vi "M03 Hybrid Car.vi"(11 "EV3 in":T1) -> (1 "Angle out":sgl, 3 "EV3 out":T1)   [LabVIEW 2016]
uses:
  <vilib>/NXT/Subs/LVHSConnector.ctl
  <vilib>/NXT/LegoClasses/BrickReference/BrickReference.lvclass
  <vilib>/NXT/Dual Mode Library/Waits/Wait_Num.vi
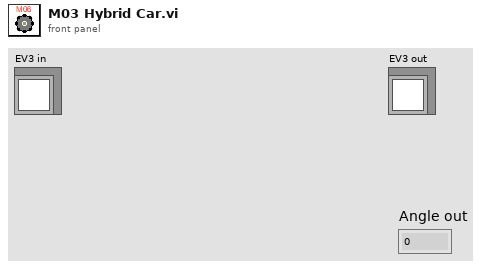
[diagram p1: front panel]
types:
  T1 = typedef "LVHSConnector.ctl" = refnum<class "BrickReference.lvclass">
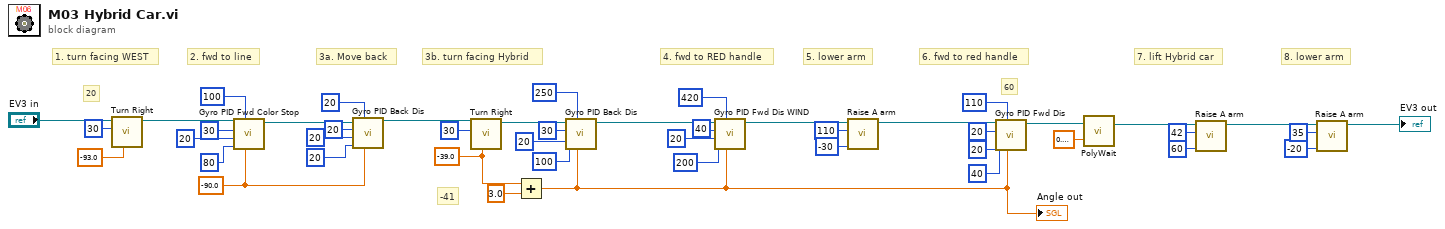
[diagram p0: block diagram]
diagram:
  w34 = sgl -39.0 ("Turning angle")
  w12 = sgl -90.0 ("Target angle")
  # "60"
  # "3a. Move back"
  # "-41"
  # "20"
  # "8. lower arm"
  # "7. lift Hybrid car"
  # "6. fwd to red handle"
  # "5. lower arm"
  # "4. fwd to RED handle"
  # "3b. turn facing Hybrid"
  # "2. fwd to line"
  # "1. turn facing WEST"
  n1 = call "Turn Right.vi"("Turning angle"=sgl -93.0, "Motor B (right)"=i8 30, "EV3 in"="EV3 in") -> ("EV3 out"=w44:T1)  [unwired: 8 in]
  n2 = call "Gyro PID Fwd Color Stop.vi"("Target angle"=w12, "Threshold to Color"=100, "Threshold to slow"=80, "Min. speed"=20, "Max. speed"=30, "EV3 in"=w44) -> ("EV3 out"=w14:T1)  [unwired: 5 in]
  n3 = call "Gyro PID Back Dis.vi"("Target angle"=w12, "Threshold to stop"=20, "Threshold to slow"=20, "Min. speed"=20, "Max. speed"=20, "EV3 in"=w14) -> ("EV3 out"=w13:T1)  [unwired: 5 in]
  n4 = call "Turn Right.vi"("Turning angle"=w34, "Motor B (right)"=i8 30, "EV3 in"=w13) -> ("EV3 out"=w7:T1)  [unwired: 8 in]
  n5 = Add(x=w34, y=sgl 3.0) -> (x+y=w2:sgl)
  "Angle out" <- w2
  n6 = call "Gyro PID Back Dis.vi"("Target angle"=w2, "Threshold to stop"=250, "Threshold to slow"=100, "Min. speed"=20, "Max. speed"=30, "EV3 in"=w7) -> ("EV3 out"=w6:T1)  [unwired: 5 in]
  n7 = call "Gyro PID Fwd Dis WIND.vi"("Target angle"=w2, "Threshold to stop"=420 ("Stop rotation"), "Threshold to slow"=200 ("Threshold to De-acc"), "Higher speed"=20, "Max. speed"=40 ("Acc"), "EV3 in"=w6) -> ("EV3 out"=w27:T1)  [unwired: 5 in]
  n8 = call "Raise A arm.vi"("Power"=i8 -30, "Rotation"=110, "EV3 in"=w27) -> ("EV3 out"=w24:T1)  [unwired: 8 in]
  n9 = call "Gyro PID Fwd Dis.vi"("Target angle"=w2, "Threshold to stop"=110, "Threshold to slow"=40, "Min. speed"=20, "Max. speed"=20, "EV3 in"=w24) -> ("EV3 out"=w20:T1)  [unwired: 5 in]
  n10 = call-poly <vilib>:"PolyWait.vi"("Time (1 sec)"=sgl 0.3, "NXT/EV3"=w20) -> ("NXT/EV3"=w21:T1)  [unwired: 2 in]
  n11 = call "Raise A arm.vi"("Power"=i8 60, "Rotation"=42, "EV3 in"=w21) -> ("EV3 out"=w16:T1)  [unwired: 8 in]
  n12 = call "Raise A arm.vi"("Power"=i8 -20, "Rotation"=35, "EV3 in"=w16) -> ("EV3 out"=→"EV3 out":T1)  [unwired: 8 in]
